vi "Set Mode (MWT) (SubVI).vi"(7 "Image Size In":T1={"Height"=3072, "Width"=3072}, 8 "REF IN":T2, 11 "Parameters In":T5={"File REF"={"AVI REF"=refnum, "DBDE REF"=refnum}, "Frame Data"={"Width"=0, "Height"=0, "Frames Per Second"=0, "Codec"=""}, "File Type"="", "Experiment Mode"=enum."Live", "Movie File Path"=path "D:/Movies Formatted on November 5th 2015/Clip (2) Formatted.raw"}) -> (0 "REF OUT":T2, 3 "Parameters Out":T5={"File REF"={"AVI REF"=refnum, "DBDE REF"=refnum}, "Frame Data"={"Width"=0, "Height"=0, "Frames Per Second"=0, "Codec"=""}, "File Type"="", "Experiment Mode"=enum."Live", "Movie File Path"=path "D:/Movies Formatted on November 5th 2015/Clip (2) Formatted.raw"}, 5 "Image Size Out":T1={"Height"=3072, "Width"=3072})   [LabVIEW 2020]
uses:
  Controls (HOST)/REF.ctl
  Controls (HOST)/Image Queue Bundle.ctl
  Controls (HOST)/Data to Disk Bundle.ctl
  Controls (HOST)/File Name Prefix.ctl
  Controls (HOST)/FPGA REF (MWT).ctl
  Controls (HOST)/Image Size.ctl
  Controls (HOST)/IMAQ Parameters.ctl
  Controls (HOST)/File REF.ctl
  <vilib>/vision/Avi.llb/IMAQ AVI2 Refnum.ctl
  Controls (HOST)/Experiment Mode.ctl
  <vilib>/Utility/error.llb/Error Cluster From Error Code.vi
  <vilib>/rvi/errors/niLvFpgaAdjustHostInterfaceError.vi
  <vilib>/rvi/interface/nirviReadWriteControl/nirviReadWriteControl.xnode
  NiFpgaLv.dll
  <vilib>/rvi/interface/Simulation/niFpgaSimulationCallBeginRW.vi
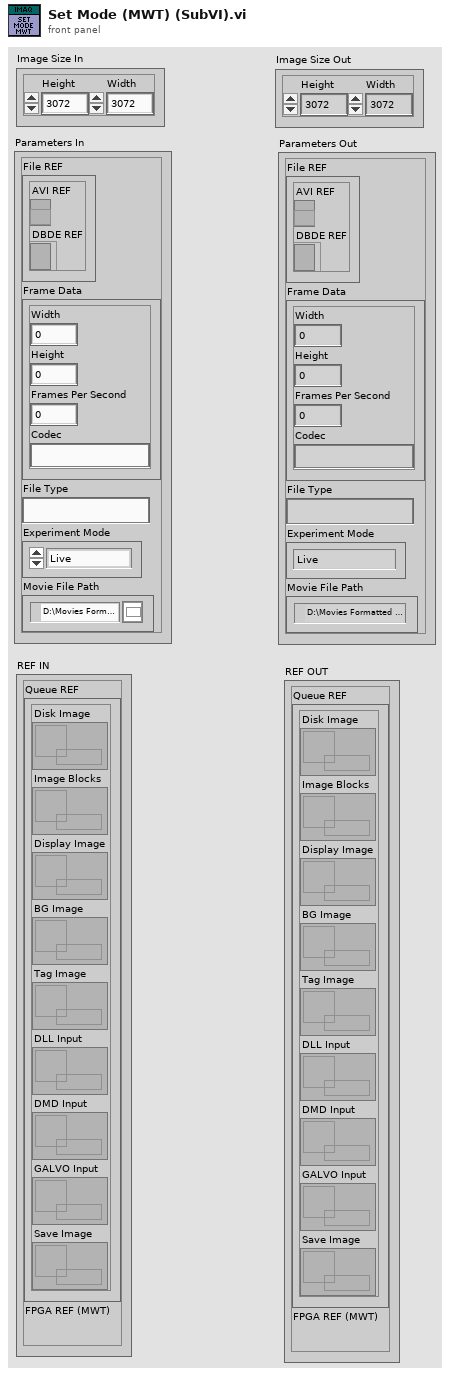
[diagram p1: front panel]
types:
  T1 = typedef "Image Size.ctl" = cluster{"Height":u16, "Width":u16}
  T2 = typedef "REF.ctl" = cluster{"Queue REF":T3, "FPGA REF (MWT)":T4}
  T3 = typedef "Image Queue Bundle.ctl" = cluster{"Disk Image":refnum<queue>, "Image Blocks":refnum<queue>, "Display Image":refnum<queue>, "BG Image":refnum<queue>, "Tag Image":refnum<queue>, "DLL Input":refnum<queue>, "DMD Input":refnum<queue>, "GALVO Input":refnum<queue>, "Save Image":refnum<queue>}
  T4 = typedef "FPGA REF (MWT).ctl" = refnum<k20>
  T5 = typedef "IMAQ Parameters.ctl" = cluster{"File REF":T6, "Frame Data":cluster{"Width":u32, "Height":u32, "Frames Per Second":u32, "Codec":string}, "File Type":string, "Experiment Mode":T8, "Movie File Path":path}
  T6 = typedef "File REF.ctl" = cluster{"AVI REF":T7, "DBDE REF":refnum<file>}
  T7 = typedef "IMAQ AVI2 Refnum.ctl" = refnum<k20>
  T8 = typedef "Experiment Mode.ctl" = enum16{"Live", "Replay"}
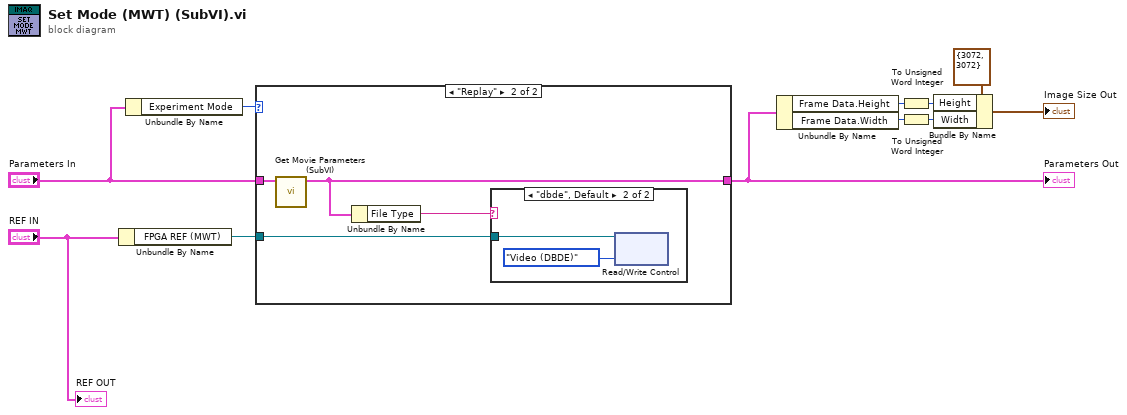
[diagram p0: block diagram]
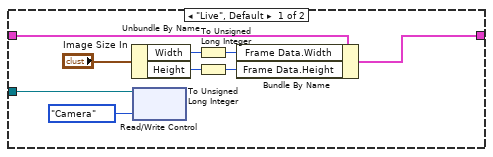
[diagram p2: hidden frame]
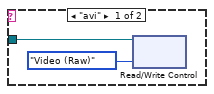
[diagram p3: hidden frame]
diagram:
  n1 = Unbundle By Name("REF IN") -> ("FPGA REF (MWT)"=w8:T4)
  n2 = Unbundle By Name("Parameters In") -> ("Experiment Mode"=w9:T8)
  n3 = case shown="\"Replay\"" w9 {
    tunnel: [w19 w23] -> w5
    tunnel: "Parameters In" -> [w20 w24]
    tunnel: w8 -> [w13 w21]
    frame "Live", Default {
      n4 = Unbundle By Name("Image Size In") -> ("Width"=w17:u16, "Height"=w16:u16)
      n5 = xnode "Read/Write Control"("FPGA VI Reference In"=w13, "Mode"=enum16{"Camera", "Video (Raw)", "Video (DBDE)"}."Camera") -> ()  [unwired: 1 in, 2 out]
      n6 = To Unsigned Long Integer(number=w17) -> (unsigned 32bit integer=w14:u32)
      n7 = To Unsigned Long Integer(number=w16) -> (unsigned 32bit integer=w15:u32)
      n8 = Bundle By Name(cluster=w20, "Frame Data.Width"=w14, "Frame Data.Height"=w15) -> (w19:T5)
    }
    frame "Replay" {
      n9 = call "Get Movie Parameters (SubVI).vi"("Parameters In"=w24) -> ("Parameters Out"=w23:T5)  [unwired: 10 in]
      n10 = Unbundle By Name(w23) -> ("File Type"=w22:string)
      n11 = case shown="\"dbde\", Default" w22 {
        tunnel: w21 -> [w25 w28]
        frame "avi" {
          n12 = xnode "Read/Write Control"("FPGA VI Reference In"=w25, "Mode"=enum16{"Camera", "Video (Raw)", "Video (DBDE)"}."Video (Raw)") -> ()  [unwired: 1 in, 2 out]
        }
        frame "dbde", Default {
          n13 = xnode "Read/Write Control"("FPGA VI Reference In"=w28, "Mode"=enum16{"Camera", "Video (Raw)", "Video (DBDE)"}."Video (DBDE)") -> ()  [unwired: 1 in, 2 out]
        }
      }
    }
  }
  "Parameters Out" <- w5
  n14 = Unbundle By Name(w5) -> ("Frame Data.Height"=w4:u32, "Frame Data.Width"=w2:u32)
  n15 = To Unsigned Word Integer(number=w4) -> (unsigned 16bit integer=w3:u16)
  n16 = To Unsigned Word Integer(number=w2) -> (unsigned 16bit integer=w1:u16)
  n17 = Bundle By Name(cluster=T1 {"Height"=3072, "Width"=3072} ("Image Size Out"), "Height"=w3, "Width"=w1) -> (→"Image Size Out":T1)
  "REF OUT" <- "REF IN"
